vi "Draw Turnos FP.vi"(10 "This VI Turnos":refnum<vi>, 11 "Sub Panel Trunos":refnum<vi>) -> ()   [LabVIEW 2020, in "Manejador Turnos.lvlib"]
uses:
  Manejador Turnos.lvlib
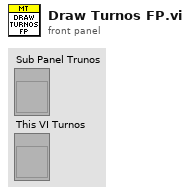
[diagram p1: front panel]
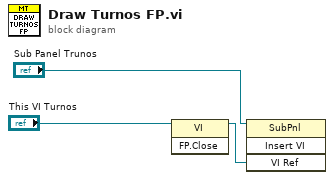
[diagram p0: block diagram]
diagram:
  n1 = invoke class="VI" method="FP.Close"(reference="This VI Turnos") -> (reference out=w3:refnum<vi>)  [unwired: 2 in, 2 out]
  n2 = invoke class="SubPnl" method="Insert VI"(reference="Sub Panel Trunos", "VI Ref"=w3) -> ()  [unwired: 2 in, 4 out]
